vi "Demodulation.vi"(2 "error in (no error)":errorcluster caption="错误输入（无错误）", 3 "delayermapdata":cdb[](array[numeric]), 4 "Qm":dbl, 5 "appended path":path) -> (0 "error IO":errorcluster, 1 "demoddata":dbl[](array[numeric]))   [LabVIEW 2015]
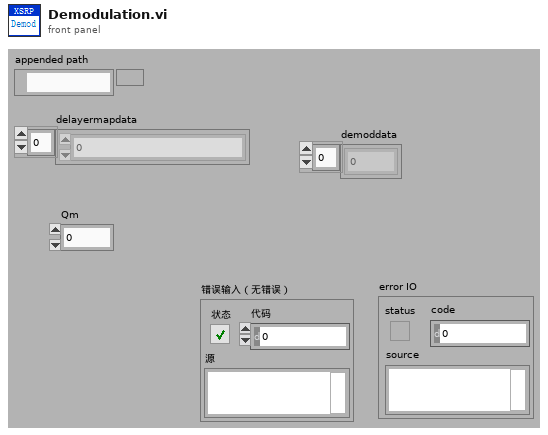
[diagram p1: front panel]
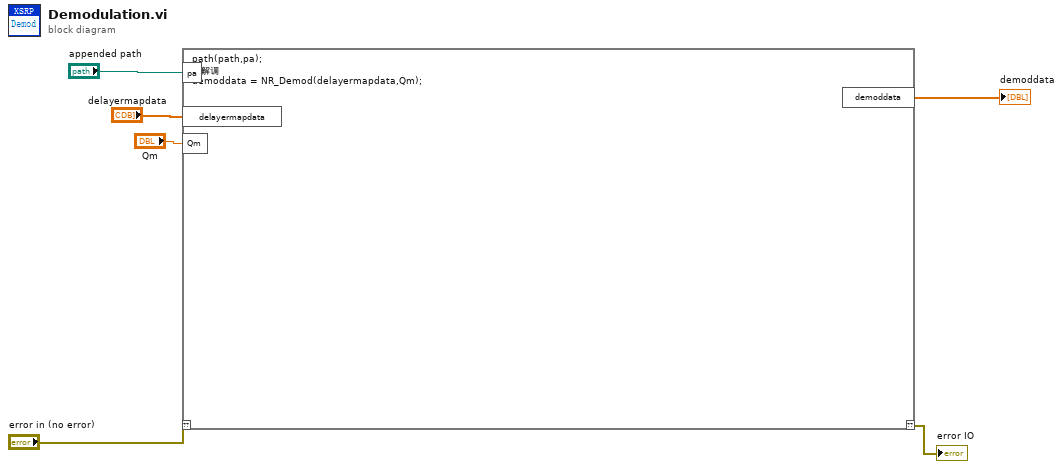
[diagram p0: block diagram]
diagram:
  n1 = script code="path(path,pa);\n%解调\ndemoddata = NR_Demod(delayermapdata,Qm);"("??"="error in (no error)", "pa"="appended path", "delayermapdata"="delayermapdata", "Qm"="Qm") -> ("??"=→"error IO":errorcluster, "demoddata"=→"demoddata":dbl[])
